vi "Last Ack Control.vi"() -> ()   [LabVIEW 2020]
uses:
  LastAck/Last Ack.lvclass
panel:
  in  "Last Ack":refnum<class "Last Ack.lvclass">
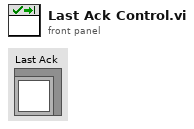
[diagram p1: front panel]
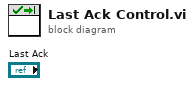
[diagram p0: block diagram]
diagram:
